vi "CRYFrequency InsDel.vi"(10 "Graph VI Ref":refnum<vi>, 11 "sAction":string) -> ()   [LabVIEW 2013]
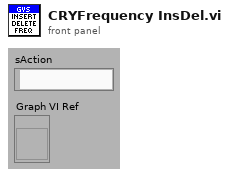
[diagram p1: front panel]
types:
  T1 = typedef "LVBoundsTypeDef.ctl" = cluster{"Width":u32, "Height":u32}
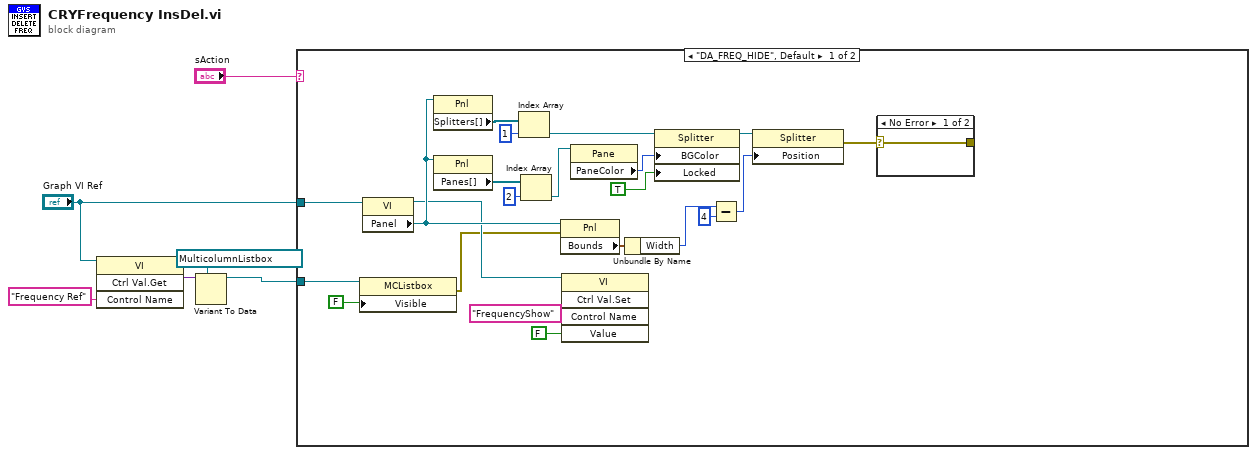
[diagram p0: block diagram]
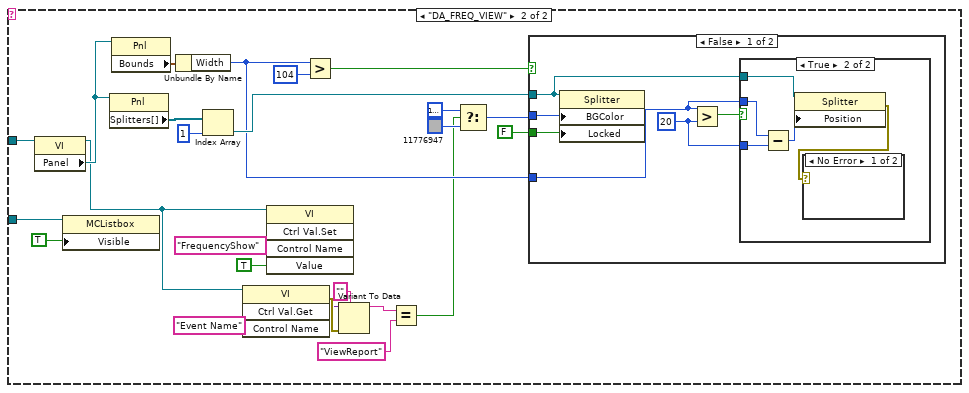
[diagram p3: hidden frame]
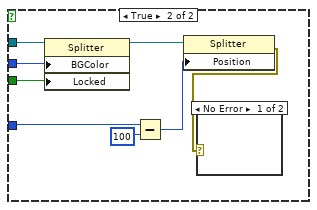
[diagram p6: hidden frame]
diagram:
  n1 = invoke class="VI" method="Ctrl Val.Get"(reference="Graph VI Ref", "Control Name"="Frequency Ref") -> ("Get Control Value Variant"=w4:variant)  [unwired: 2 in, 3 out]
  n2 = Variant To Data(type=refnum<vi> refnum ("GMListbox"), Variant=w4) -> (data=w1:refnum<vi>)  [unwired: 1 in, 1 out]
  n3 = case shown="\"DA_FREQ_HIDE\", Default" "sAction" {
    tunnel: "Graph VI Ref" -> [w11 w51]
    tunnel: w1 -> [w27 w45]
    frame "DA_FREQ_HIDE", Default {
      n4 = property class="MCListbox"(reference=w27, "Visible"=FALSE) -> (error out=w7:errorcluster)  [unwired: 1 in, 1 out]
      n5 = property class="VI"(reference=w11) -> (reference out=w8:refnum<vi>, "Panel"=w21:refnum<vi>)  [unwired: 1 in, 1 out]
      n6 = property class="Pnl"(reference=w21) -> ("Splitters[]"=w14:refnum<vi>[])  [unwired: 1 in, 2 out]
      n7 = property class="Pnl"(reference=w21) -> ("Panes[]"=w12:refnum<vi>[])  [unwired: 1 in, 2 out]
      n8 = Index Array(array=w14, index=1) -> (element=w15:refnum<vi>)
      n9 = Index Array(array=w12, index=2) -> (element=w18:refnum<vi>)
      n10 = property class="Pnl"(reference=w21, error in=w7) -> ("Bounds"=w22:T1)  [unwired: 2 out]
      n11 = invoke class="VI" method="Ctrl Val.Set"(reference=w8, "Control Name"="FrequencyShow", "Value"=FALSE ("Visible")) -> ()  [unwired: 2 in, 5 out]
      n12 = property class="Pane"(reference=w18) -> ("PaneColor"=w16:u32)  [unwired: 1 in, 2 out]
      n13 = Unbundle By Name(w22) -> ("Width"=w23:u32)
      n14 = property on="Property Node" class="Splitter"(reference=w15, "BGColor"=w16, "Locked"=TRUE ("Splitter Position Locked")) -> (reference out=w19:refnum<vi>)  [unwired: 1 in, 1 out]
      n15 = Subtract(x=w23, y=u32 4) -> (x-y=w25:u32)
      n16 = property on="Property Node" class="Splitter"(reference=w19, "Position"=w25) -> (error out=w20:errorcluster)  [unwired: 1 in, 1 out]
      n17 = case shown="No Error" w20 {
        selector: w20 -> [w29 w30]
        tunnel: [w29 w30] -> _
        frame No Error {
        }
        frame Error {
        }
      }
    }
    frame "DA_FREQ_VIEW" {
      n18 = property class="VI"(reference=w51) -> (reference out=w37:refnum<vi>, "Panel"=w53:refnum<vi>)  [unwired: 1 in, 1 out]
      n19 = property class="MCListbox"(reference=w45, "Visible"=TRUE) -> ()  [unwired: 1 in, 2 out]
      n20 = property class="Pnl"(reference=w53) -> ("Splitters[]"=w55:refnum<vi>[])  [unwired: 1 in, 2 out]
      n21 = property class="Pnl"(reference=w53) -> ("Bounds"=w52:T1)  [unwired: 1 in, 2 out]
      n22 = Unbundle By Name(w52) -> ("Width"=w46:u32)
      n23 = Index Array(array=w55, index=1) -> (element=w48:refnum<vi>)
      n24 = invoke class="VI" method="Ctrl Val.Get"(reference=w37, "Control Name"="Event Name") -> (error out=w39:errorcluster, "Get Control Value Variant"=w38:variant)  [unwired: 2 in, 2 out]
      n25 = invoke class="VI" method="Ctrl Val.Set"(reference=w37, "Control Name"="FrequencyShow", "Value"=TRUE ("Visible")) -> ()  [unwired: 2 in, 5 out]
      n26 = Greater?(x=w46, y=u32 104) -> (0:w49:bool)
      n27 = Variant To Data(error in=w39, type="" ("Control Name"), Variant=w38) -> (data=w36:string)  [unwired: 1 out]
      n28 = Equal?(x=w36, y="ViewReport" ("Control Name")) -> (x = y?=w32:bool)
      n29 = Select(t=u32 16777226, s=w32, f=u32 11776947) -> (s? t:f=w33:u32)
      n30 = case shown="False" w49 {
        tunnel: w48 -> [w58 w72]
        tunnel: w33 -> [w61 w73]
        tunnel: FALSE ("Splitter Position Locked") -> [w60 w74]
        tunnel: w46 -> [w57 w70]
        frame False {
          w56 = u32 20 ("y")
          n31 = property on="Property Node" class="Splitter"(reference=w58, "BGColor"=w61, "Locked"=w60) -> ()  [unwired: 1 in, 2 out]
          n32 = Greater?(x=w57, y=w56) -> (0:w59:bool)
          n33 = case shown="True" w59 {
            tunnel: w58 -> [_ w66]
            tunnel: w57 -> [_ w65]
            tunnel: w56 -> [_ w63]
            frame False {
            }
            frame True {
              n34 = Subtract(x=w65, y=w63) -> (x-y=w64:u32)
              n35 = property on="Property Node" class="Splitter"(reference=w66, "Position"=w64) -> (error out=w62:errorcluster)  [unwired: 1 in, 1 out]
              n36 = case shown="No Error" w62 {
                frame No Error {
                }
                frame Error {
                }
              }
            }
          }
        }
        frame True {
          n37 = property on="Property Node" class="Splitter"(reference=w72, "BGColor"=w73, "Locked"=w74) -> (reference out=w68:refnum<vi>)  [unwired: 1 in, 1 out]
          n38 = Subtract(x=w70, y=u32 100) -> (x-y=w69:u32)
          n39 = property on="Property Node" class="Splitter"(reference=w68, "Position"=w69) -> (error out=w67:errorcluster)  [unwired: 1 in, 1 out]
          n40 = case shown="No Error" w67 {
            frame No Error {
            }
            frame Error {
            }
          }
        }
      }
    }
  }
